vi "get_PID.vi"(0 "heat_board_control in":refnum<class "heat_board_control.lvclass">, 11 "error in (no error)":errorcluster) -> (4 "heat_board_control out":refnum<class "heat_board_control.lvclass">, 6 "Cluster":T1, 15 "error out":errorcluster)   [LabVIEW 2015, in "heat_board_control.lvclass"]
uses:
  heat_board_control.lvclass
  heat_board_control.lvclass/heat_board_control.ctl
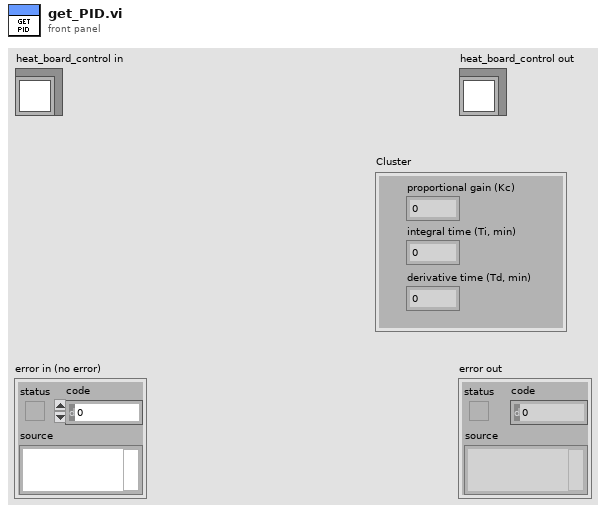
[diagram p1: front panel]
types:
  T1 = cluster{"proportional gain (Kc)":dbl, "derivative time (Td, min)":dbl, "integral time (Ti, min)":dbl}
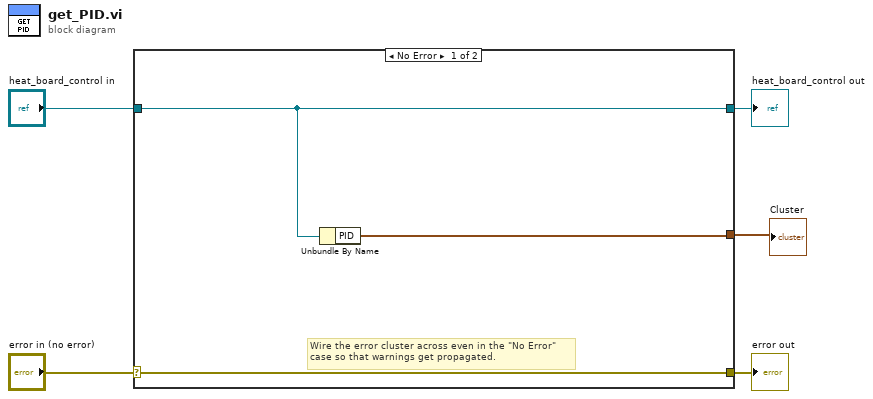
[diagram p0: block diagram]
diagram:
  n1 = case shown="No Error" "error in (no error)" {
    selector: "error in (no error)" -> [w8 w10]
    tunnel: [w8 w10] -> w4
    tunnel: [w7 w9] -> w2
    tunnel: "heat_board_control in" -> [w7 w9]
    tunnel: [w6 _] -> w1
    frame No Error {
      # "Wire the error cluster across even in the \"No Error\"\ncase so that warnings get propagated."
      n2 = Unbundle By Name(w7) -> ("PID"=w6:cluster{"P":dbl, "I":dbl, "D":dbl})
    }
    frame Error {
    }
  }
  "error out" <- w4
  "heat_board_control out" <- w2
  "Cluster" <- w1
